vi "Build Tags from JSON List.vi"(8 "error in (no error)":errorcluster, 10 "JSON Config String":string) -> (0 "error out":errorcluster)   [LabVIEW 2020, in "Tag Engine.lvlib"]
doc: "Build multiple Tags from a JSON array of Tag configurations."
uses:
  Tag Engine.lvlib
  <vilib>/JDP Science/JSONtext/JSONtext.lvlib
panel:
  # "Expecting an array of Tag Configurations in JSON format"
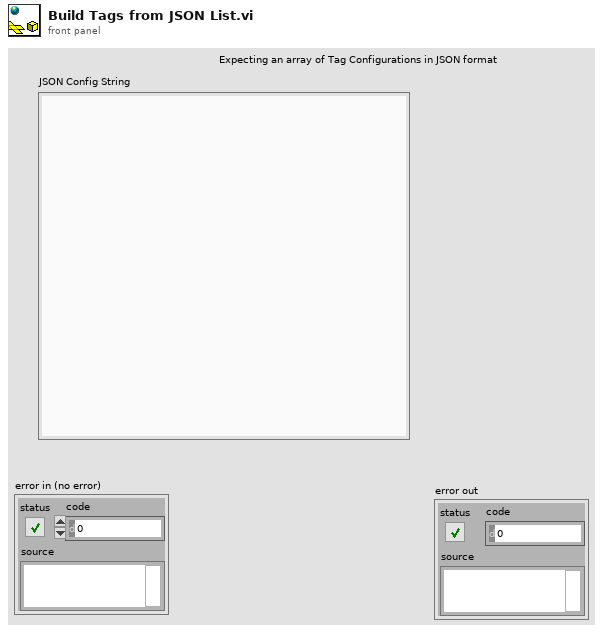
[diagram p1: front panel]
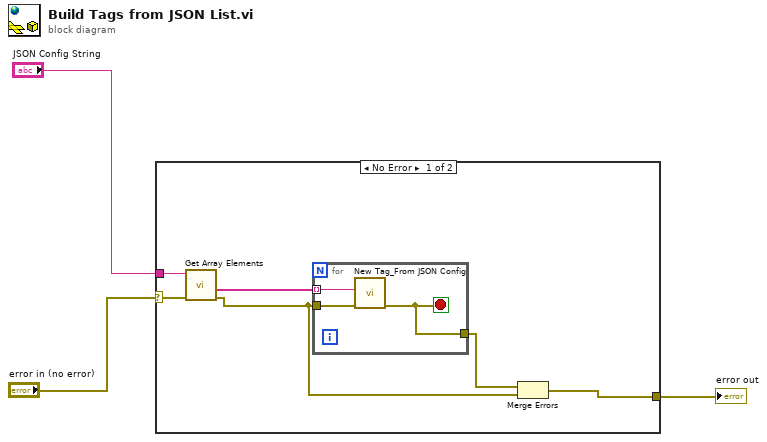
[diagram p0: block diagram]
diagram:
  n1 = case shown="No Error" "error in (no error)" {
    selector: "error in (no error)" -> [w7 w13]
    tunnel: "JSON Config String" -> [w9 _]
    tunnel: [w4 w13] -> w2
    frame No Error {
      n2 = call <vilib>:"Get Array Elements.vi"("error in (no error)"=w7, "JSON"=w9) -> ("error out"=w6:errorcluster, "<JSON>"=w8:string[])  [unwired: 7 in, 1 out]
      n3 = for {
        tunnel: w8 -> [w12] mode=indexing
        tunnel: [w11] -> w5
        tunnel: w6 -> [w10]
        stop <- w11 stop-if-true
        n4 = call "New Tag_From JSON Config.vi"("error in (no error)"=w10, "JSON Tag Config"=w12) -> ("error out"=w11:errorcluster)  [unwired: 8 in, 1 out]
      }
      n5 = Merge Errors(w5, w6) -> (w4:errorcluster)
    }
    frame Error {
    }
  }
  "error out" <- w2
